vi "NewExperimentDialog.vi"(8 "error in (no error)":errorcluster) -> (0 "error out":errorcluster, 1 "Goal 2":string, 2 "File Path 2":path=path "E:/LINKAM Measurements_Naama/200514", 3 "Experiment Name 2":string="t", 4 "Add Entry Pressed?":bool=TRUE)   [LabVIEW 2015]
doc: "Use this template to build a VI to use as a subVI."
uses:
  SettingsEnum.ctl
panel:
  in  "Get focus":string
  in  "Goal":string
  in  "File Path":path=path "E:/LINKAM Measurements_Naama"
  in  "Experiment Name":string
  in  "Cancel Button":bool
  in  "Add Entry Button":bool
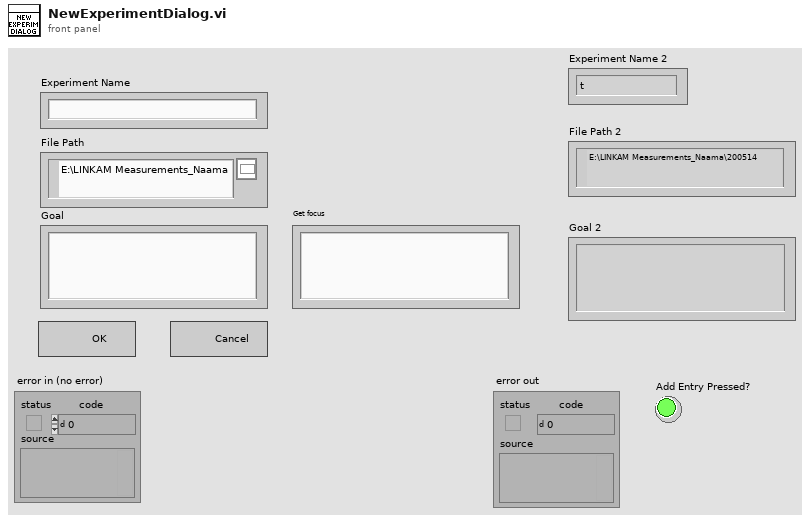
[diagram p1: front panel]
types:
  T1 = typedef "SettingsEnum.ctl" = enum16{"Set Mag Type", "Get Mag Type", "Get System Name", "Set System Name", "Set Ramp Path", "Set Main Path", "Get Ramp Path", "Set All Data", "Get Main Path", "Init"}
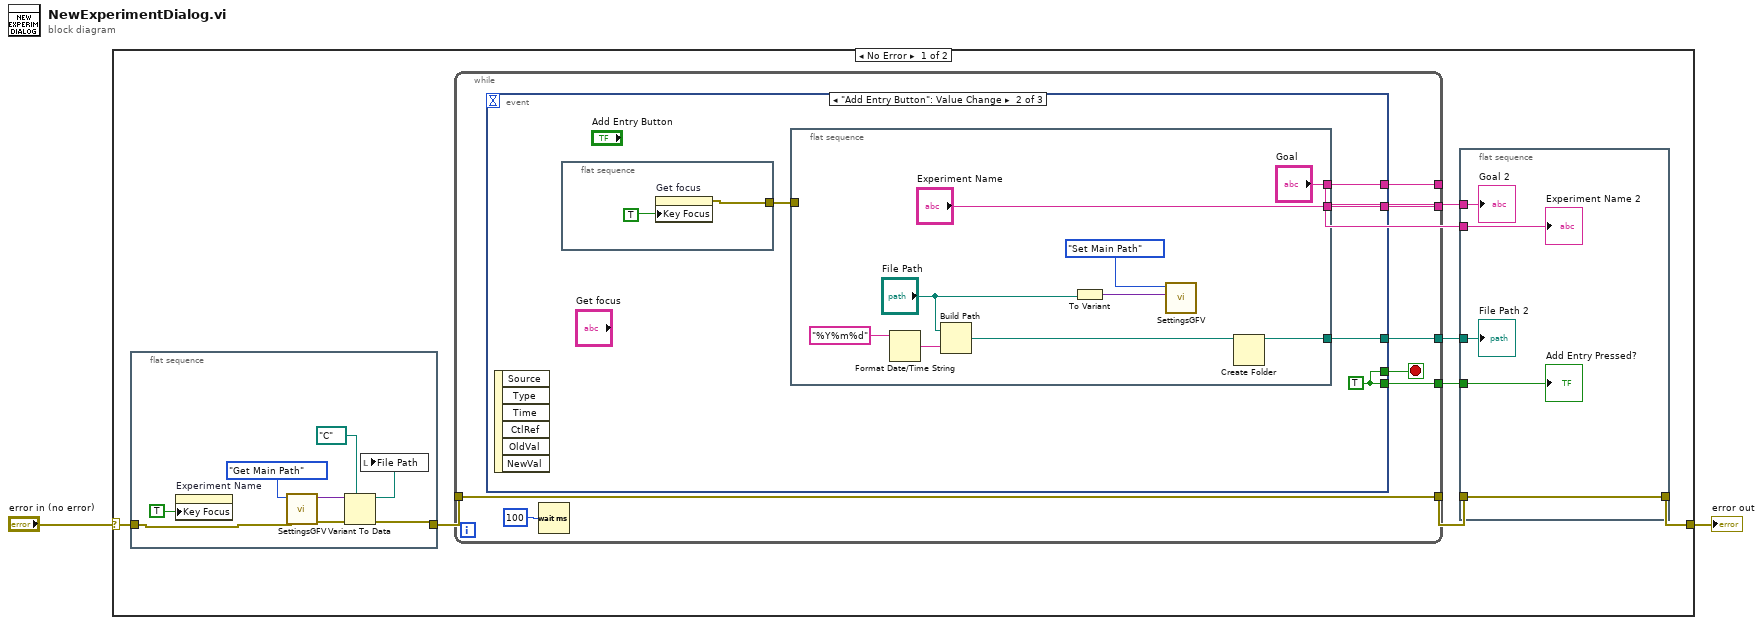
[diagram p0: block diagram]
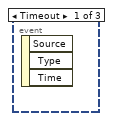
[diagram p2: hidden frame]
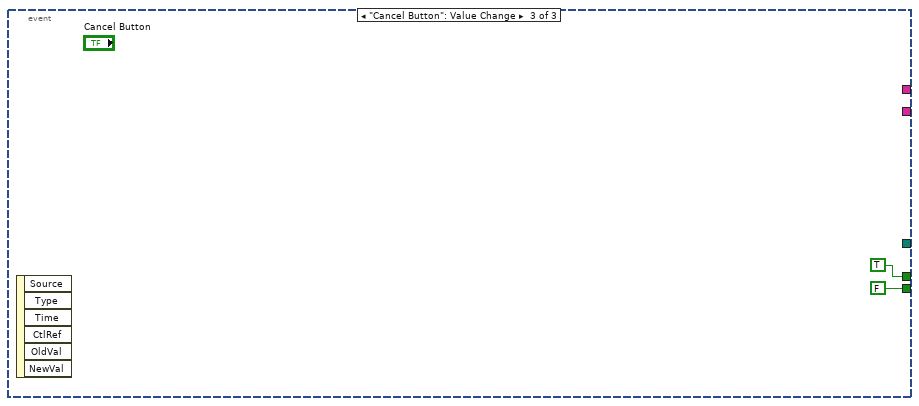
[diagram p3: hidden frame]
diagram:
  n1 = case shown="No Error" "error in (no error)" {
    selector: "error in (no error)" -> [w6 w49]
    tunnel: [w4 w49] -> w1
    frame No Error {
      n2 = flat-sequence {
        tunnel: w6 -> [w18]
        tunnel: [w17] -> w5
        frame #0 {
          n3 = property on="Experiment Name" class="Str"("Key Focus"=TRUE) -> ()  [unwired: 2 in, 2 out]
          n4 = call "SettingsGFV.vi"("error in (no error)"=w18, "Enum"=SettingsEnum."Get Main Path") -> ("error out"=w19:errorcluster, "Variant Output"=w22:variant)  [unwired: 8 in]
          n5 = Variant To Data(error in=w19, type=path "C:/" ("default value"), Variant=w22) -> (data=w16:path, error out=w17:errorcluster)
          n6 = local write "File Path"(w16) -> ()
        }
      }
      n7 = while {
        tunnel: [w29] -> w10
        tunnel: [w27] -> w9
        tunnel: [w26] -> w8
        tunnel: [w25] -> w7
        tunnel: w5 -> [w24]
        tunnel: [w24] -> w3
        stop <- w30 stop-if-true
        n8 = event shown="[1] \"Add Entry Button\": Value Change" {
          selector: _ -> [_ _ _]
          dyn-events: _ -> [_ _ _]
          timeout: _ -> [_ _ _]
          tunnel: [_ w35 TRUE] -> w30
          tunnel: [_ w35 FALSE] -> w29
          tunnel: [_ w34 _] -> w27
          tunnel: [_ w32 _] -> w26
          tunnel: [_ w33 _] -> w25
          event Timeout {
            n9 = event-data() -> ()  [unwired: 1 in, 3 out]
          }
          event "Add Entry Button": Value Change {
            w35 = TRUE
            n10 = event-data() -> ()  [unwired: 1 in, 6 out]
            n11 = flat-sequence {
              tunnel: [w37] -> w31
              frame #0 {
                n12 = property on="Get focus" class="Str"("Key Focus"=TRUE) -> (error out=w37:errorcluster)  [unwired: 2 in, 1 out]
              }
            }
            n13 = flat-sequence {
              tunnel: ["Experiment Name"] -> w34
              tunnel: ["Goal"] -> w33
              tunnel: [w42] -> w32
              tunnel: w31 -> [_]
              frame #0 {
                n14 = Format Date/Time String(time format string (%c)="%Y%m%d") -> (date/time string=w43:string)  [unwired: 2 in]
                n15 = Build Path(base path="File Path", name or relative path=w43) -> (appended path=w41:path)
                n16 = To Variant(anything="File Path") -> (Variant=w39:variant)
                n17 = call "SettingsGFV.vi"("Variant Input"=w39, "Enum"=SettingsEnum."Set Main Path") -> ()  [unwired: 8 in, 2 out]
                n18 = Create Folder(path (use dialog)=w41) -> (created path=w42:path)  [unwired: 2 in, 2 out]
              }
            }
          }
          event "Cancel Button": Value Change {
            n19 = event-data() -> ()  [unwired: 1 in, 6 out]
          }
        }
        n20 = Wait (ms)(milliseconds to wait=u32 100) -> ()  [unwired: 1 out]
      }
      n21 = flat-sequence {
        tunnel: w10 -> [w15]
        tunnel: w9 -> [w14]
        tunnel: w8 -> [w13]
        tunnel: w7 -> [w12]
        tunnel: w3 -> [w11]
        tunnel: [w11] -> w4
        frame #0 {
          "Add Entry Pressed?" <- w15
          "Experiment Name 2" <- w14
          "File Path 2" <- w13
          "Goal 2" <- w12
        }
      }
    }
    frame Error {
    }
  }
  "error out" <- w1
